vi "ReadWrite_Text.vi"(0 "file path":path=path "C:/Projects/labview_tips_2024/src/Assessment01/TextFile.txt", 5 "Write String":string, 11 "error in":errorcluster, 13 "Read/Write":enum16{"Read", "Write"}(ring)) -> (4 "Read String":string, 15 "error out":errorcluster)   [LabVIEW 2023, in "Unit Testing CA1.lvlib"]
uses:
  Unit Testing CA1.lvlib
  <vilib>/Utility/error.llb/Trim Whitespace One-Sided.vi
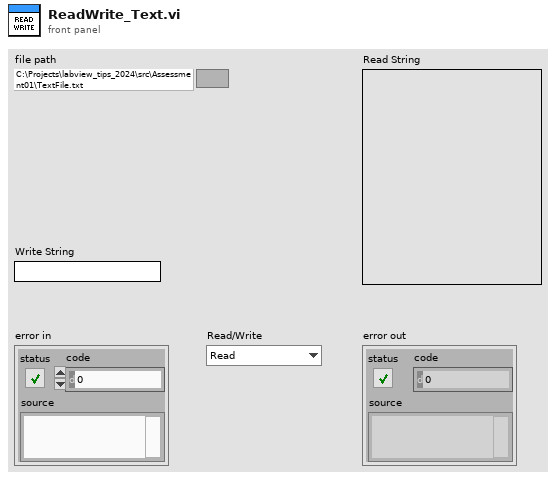
[diagram p1: front panel]
types:
  T1 = enum16{"open", "replace", "create", "open or create", "replace or create", "replace or create with confirmation"}
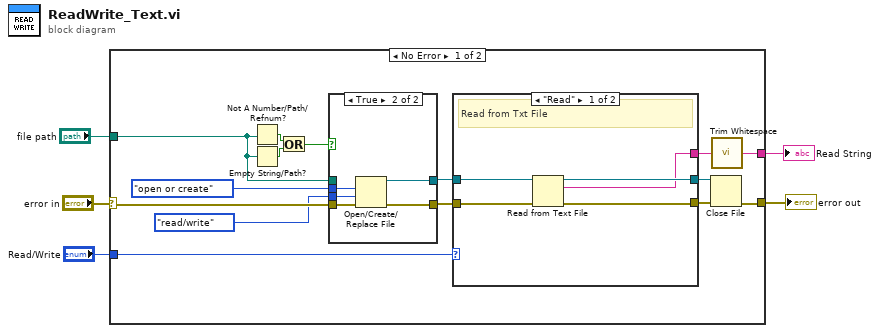
[diagram p0: block diagram]
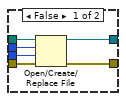
[diagram p2: hidden frame]
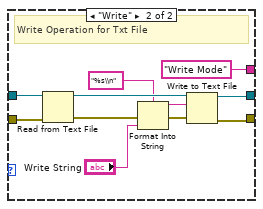
[diagram p3: hidden frame]
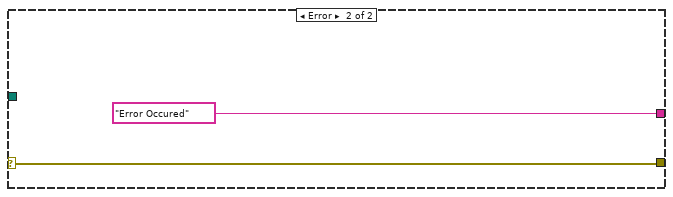
[diagram p4: hidden frame]
diagram:
  n1 = case shown="No Error" "error in" {
    selector: "error in" -> [w13 w49]
    tunnel: [w20 w49] -> w4
    tunnel: [w6 "Error Occured"] -> w3
    tunnel: "file path" -> [w8 _]
    tunnel: "Read/Write" -> [w7 _]
    frame No Error {
      n2 = Not A Number/Path/Refnum?(number/path/refnum=w8) -> (NaN/Path/Refnum?=w15:bool)
      n3 = Empty String/Path?(string/path=w8) -> (empty?=w14:bool)
      n4 = Or(x=w15, y=w14) -> (x .or. y?=w16:bool)
      n5 = case shown="True" w16 {
        tunnel: w13 -> [w26 w30]
        tunnel: [w25 w31] -> w9
        tunnel: [w24 w29] -> w10
        tunnel: w8 -> [w23 _]
        tunnel: T1."open or create" ("operation (0:open)") -> [w22 w28]
        tunnel: enum16{"read/write", "read-only", "write-only"}."read/write" ("access (0:read/write)") -> [w21 w27]
        frame False {
          n6 = Open/Create/Replace File(file path (use dialog)=w23, error in=w26, operation (0:open)=w22, access (0:read/write)=w21) -> (refnum out=w24:refnum<file>, error out=w25:errorcluster)  [unwired: 2 in, 1 out]
        }
        frame True {
          n7 = Open/Create/Replace File(error in=w30, operation (0:open)=w28, access (0:read/write)=w27) -> (refnum out=w29:refnum<file>, error out=w31:errorcluster)  [unwired: 3 in, 1 out]
        }
      }
      n8 = case shown="\"Read\"" w7 {
        tunnel: w10 -> [w36 w42]
        tunnel: w9 -> [w35 w45]
        tunnel: [w32 "Write Mode"] -> w17
        tunnel: [w34 w44] -> w19
        tunnel: [w33 w47] -> w18
        frame "Read" {
          # "Read from Txt File"
          n9 = Read from Text File(file (use dialog)=w36, error in=w35) -> (refnum out=w33:refnum<file>, text=w32:string, error out=w34:errorcluster)  [unwired: 2 in, 1 out]
        }
        frame "Write" {
          # "Write Operation for Txt File"
          n10 = Read from Text File(file (use dialog)=w42, error in=w45) -> (refnum out=w43:refnum<file>, error out=w40:errorcluster)  [unwired: 2 in, 2 out]
          n11 = Format Into String(format string="%s\\n", error in=w40, "Write String") -> (resulting string=w38:string, error out=w39:errorcluster)  [unwired: 1 in]
          n12 = Write to Text File(file (use dialog)=w43, text=w38, error in=w39) -> (refnum out=w47:refnum<file>, error out=w44:errorcluster)  [unwired: 1 in, 1 out]
        }
      }
      n13 = Close File(refnum=w18, error in=w19) -> (error out=w20:errorcluster)  [unwired: 1 out]
      n14 = call <vilib>:"Trim Whitespace.vi"("string"=w17) -> ("trimmed string"=w6:string)  [unwired: 1 in]
    }
    frame Error {
    }
  }
  "error out" <- w4
  "Read String" <- w3
